vi "collect_allLT_img.vi"() -> (0 "cts/sec":dbl, 1 "counts":i32)   [LabVIEW 2015]
uses:
  phlib.dll
panel:
  out "counts per\niteration":i32[](array[numeric])
  out "iterations":i32
  out "index of element":i32
  out "okay":bool
  out "trunc buffer":u32[](array[numeric]) format="%08x"
  out "buffer":u32[](array[numeric]) format="%08x"
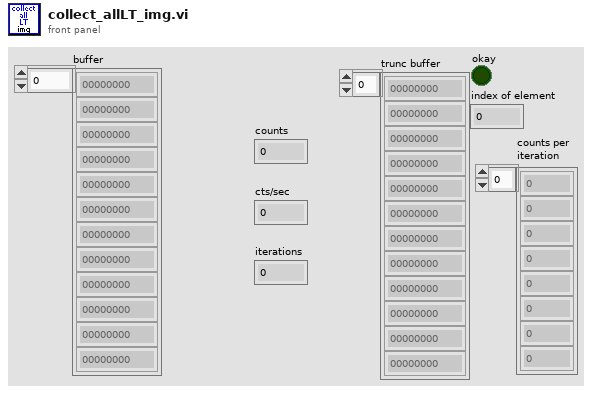
[diagram p1: front panel]
types:
  T1 = cluster{"initialized":bool, "devidx":i32, "Ch0 Level":i32, "Ch0 ZeroX":i32, "Ch1 Level":i32, "Ch1 ZeroX":i32, "sync rate":i32, "resolution":i32, "acq time":i32, "acq rate":i32, "# bins":u32, "Bin size":enum16{"1", "2", "4", "8", "16", "32", "64", "128"}, "min photons":u32, "truncate":u32}
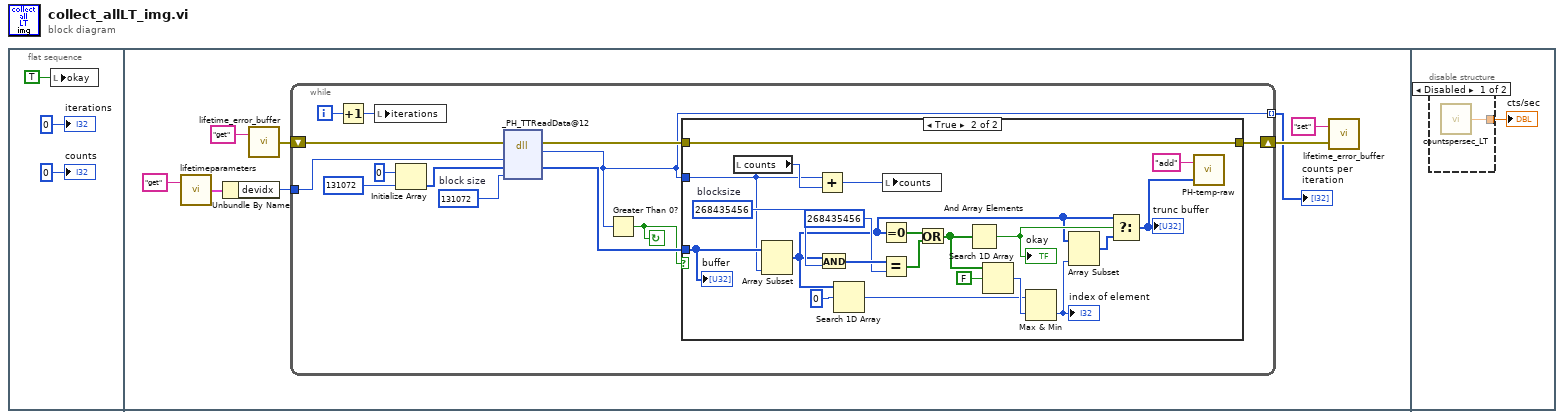
[diagram p0: block diagram]
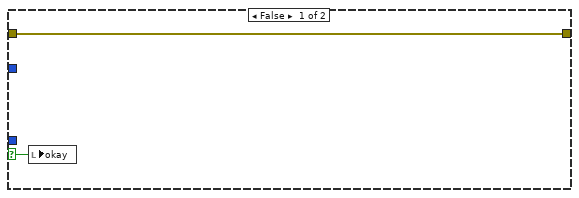
[diagram p2: hidden frame]
diagram:
  n1 = flat-sequence {
    frame #0 {
      n2 = local write "okay"(TRUE ("okay")) -> ()
      "counts" <- 0 ("iterations")
      "iterations" <- 0 ("iterations")
    }
    frame #1 {
      n3 = call "lifetimeparameters.vi"("command"="get") -> ("Params out"=w8:T1)  [unwired: 1 in]
      n4 = Unbundle By Name(w8) -> ("devidx"=w7:i32)
      n5 = call "lifetime_error_buffer.vi"("command"="get") -> ("error out"=w10:errorcluster)  [unwired: 1 in]
      n6 = while {
        tunnel: w7 -> [w14]
        shift-right: [w15] -> w5
        shift-left: w10 -> [w18]
        tunnel: [w12] -> w4 mode=indexing
        i -> [w17]
        stop <- w13 continue-if-true
        w20 = 131072  # block size
        n7 = Increment(x=w17) -> (x+1=w19:i32)
        n8 = local write "iterations"(w19) -> ()
        n9 = Initialize Array(u32 0, 131072) -> (w22:u32[])
        n10 = dll-call lib="phlib.dll" fn="_PH_TTReadData@12" label="PH_TTReadData"(error in=w18, "devidx"=w14, "buffer"=w22, "blocksize"=w20) -> (error out=w16:errorcluster, "return type"=w12:i32, "buffer"=w21:u32[])  [unwired: 4 in, 1 out]
        n11 = Greater Than 0?(x=w12) -> (x > 0?=w13:bool)
        n12 = case shown="True" w13 {
          selector: w13 -> [w25 _]
          tunnel: w21 -> [_ w29]
          tunnel: w12 -> [_ w28]
          tunnel: w16 -> [w26 w45]
          tunnel: [w26 w45] -> w15
          frame False {
            n13 = local write "okay"(w25) -> ()
          }
          frame True {
            w34 = u32 268435456  # blocksize
            n14 = local read "counts"() -> (w46:i32)
            n15 = Array Subset(array=w29, length=w28) -> (w27:u32[])  [unwired: 1 in]
            n16 = Add(x=w28, y=w46) -> (x+y=w47:i32)
            n17 = And(x=w27, y=w34) -> (x .and. y?=w36:u32[])
            n18 = Search 1D Array(1D array=w27, element=u32 0) -> (index of element=w43:i32)  [unwired: 1 in]
            n19 = Equal To 0?(x=w27) -> (x = 0?=w38:bool[])
            n20 = Equal?(x=w36, y=u32 268435456 ("blocksize")) -> (x = y?=w37:bool[])
            n21 = local write "counts"(w47) -> ()
            n22 = Or(x=w38, y=w37) -> (x .or. y?=w40:bool[])
            n23 = And Array Elements(Boolean array=w40) -> (logical AND=w39:bool)
            "okay" <- w39
            n24 = Search 1D Array(1D array=w40, element=FALSE) -> (index of element=w44:i32)  [unwired: 1 in]
            n25 = Max & Min(x=w43, y=w44) -> (min(x,y)=w30:i32)  [unwired: 1 out]
            "index of element" <- w30
            n26 = Array Subset(array=w27, length=w30) -> (w31:u32[])  [unwired: 1 in]
            n27 = Select(t=w27, s=w39, f=w31) -> (s? t:f=w32:u32[])
            "trunc buffer" <- w32
            n28 = call "PH-temp-raw.vi"("array in"=w32, "command"="add") -> ()  [unwired: 1 out]
            "buffer" <- w29
          }
        }
      }
      "counts per\niteration" <- w4
      n29 = call "lifetime_error_buffer.vi"("error in"=w5, "command"="set") -> ()  [unwired: 1 out]
    }
    frame #2 {
      n30 = disable-structure shown="Disabled" {
        disable-tunnel: [w49 _] -> w48
        frame Disabled {
          n31 = call "countspersec_LT.vi"() -> ("Avg cts/s"=w49:dbl)
        }
        frame Enabled {
        }
      }
      "cts/sec" <- w48
    }
  }
